vi "Get State Aliases from Case Structure Frame Name.vi"(8 "error in (no error)":errorcluster, 11 "Frame or State Name":string) -> (0 "error out":errorcluster, 2 "Event Frame?":bool, 3 "State Aliases":string[](array[string]))   [LabVIEW 2013]
uses:
  <userlib>/_OpenG.lib/string/string.llb/Trim Whitespace (String)__ogtk.vi
  <userlib>/_OpenG.lib/array/array.llb/Filter 1D Array with Scalar (String)__ogtk.vi
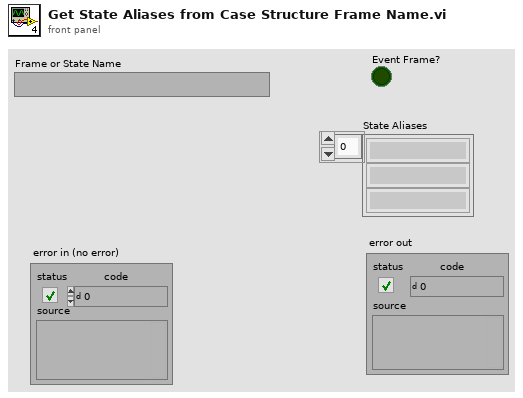
[diagram p1: front panel]
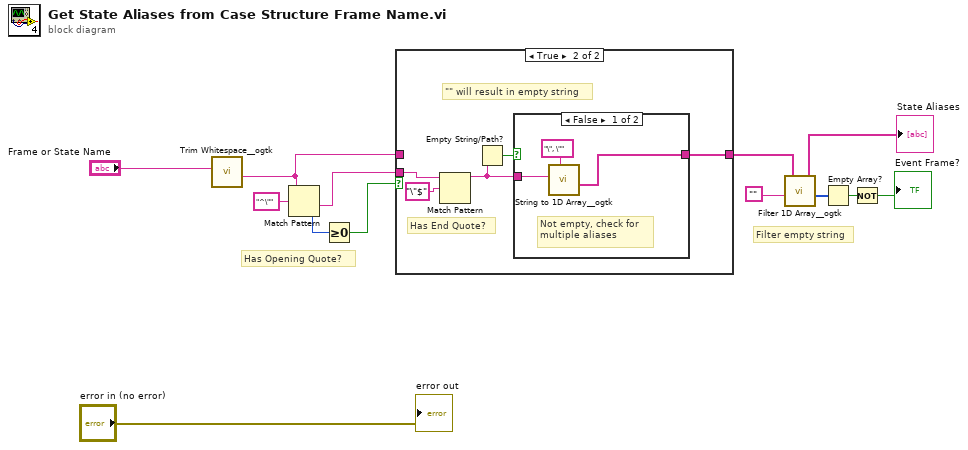
[diagram p0: block diagram]
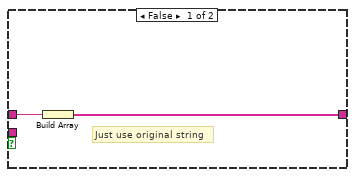
[diagram p2: hidden frame]
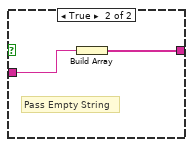
[diagram p3: hidden frame]
diagram:
  # "Filter empty string"
  # "Has Opening Quote?"
  n1 = call-poly <userlib>:"Trim Whitespace__ogtk.vi"("String in"="Frame or State Name") -> ("String out"=w8:string)  [unwired: 6 in]
  n2 = Match Pattern(string=w8, regular expression="^\"") -> (after substring=w9:string, offset past match=w11:i32)  [unwired: 1 in, 2 out]
  n3 = Greater Or Equal To 0?(x=w11) -> (x >= 0?=w10:bool)
  n4 = case shown="True" w10 {
    tunnel: [w15 w20] -> w3
    tunnel: w9 -> [_ w18]
    tunnel: w8 -> [w14 _]
    frame False {
      # "Just use original string"
      n5 = Build Array(w14) -> (w15:string[])
    }
    frame True {
      # "\"\" will result in empty string"
      # "Has End Quote?"
      n6 = Match Pattern(string=w18, regular expression="\"$") -> (before substring=w17:string)  [unwired: 1 in, 3 out]
      n7 = Empty String/Path?(string/path=w17) -> (empty?=w16:bool)
      n8 = case shown="False" w16 {
        tunnel: [w22 w24] -> w20
        tunnel: w17 -> [w21 w25]
        frame False {
          # "Not empty, check for\nmultiple aliases"
          n9 = call <userlib>:"String to 1D Array__ogtk.vi"("delimiter (Tab)"="\", \"", "string"=w21) -> ("Array of Strings"=w22:string[])  [unwired: 9 in]
        }
        frame True {
          # "Pass Empty String"
          n10 = Build Array(w25) -> (w24:string[])
        }
      }
    }
  }
  n11 = call-poly <userlib>:"Filter 1D Array__ogtk.vi"("items to filter"="", "array"=w3) -> ("filtered item indices"=w6:i32[], "filtered array"=→"State Aliases":string[])  [unwired: 4 in]
  n12 = Empty Array?(array=w6) -> (empty?=w5:bool)
  n13 = Not(x=w5) -> (.not. x?=→"Event Frame?":bool)
  "error out" <- "error in (no error)"
